vi "Lvi Subsystem Set Channel Gain.vi"(8 "error in (no error)":errorcluster, 9 "Gain":dbl, 10 "Channel":u32, 11 "TaskRef":i32) -> (0 "error out":errorcluster, 1 "Gain out":dbl, 2 "function return":u32(ring), 3 "TaskRef out":i32)   [LabVIEW 2022 SP3, in "DtLvLink.lvlib"]
doc: "Calls directly into the entry points of the DLL of the Data Acq SDK to specify the gain of a virtual channel for the specified task. This VI is used by the higher-level VI, DtOLSetChanGain."
uses:
  DtLvLink.lvlib
  <userlib>/LV-Link3/DtLvLink_64.dll
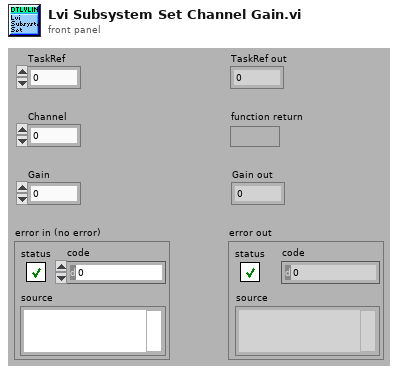
[diagram p1: front panel]
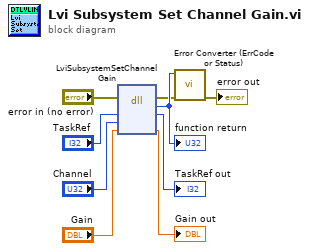
[diagram p0: block diagram]
diagram:
  n1 = dll-call lib="C:/Program Files/National Instruments/LabVIEW 2022/user.lib/LV-Link3/DtLvLink_64.*" fn="LviSubsystemSetChannelGain"(error in="error in (no error)", "TaskRef"="TaskRef", "Channel"="Channel", "Gain"="Gain") -> (error out=w3:errorcluster, "return type"=w9:u32, "TaskRef"=→"TaskRef out":i32, "Gain"=→"Gain out":dbl)  [unwired: 3 in, 1 out]
  "function return" <- w9
  n2 = call "Error Converter (ErrCode or Status).vi"("error in (no error)"=w3, "error code"=w9) -> ("error out"=→"error out":errorcluster)  [unwired: 9 in]
